vi "WM NH Extreme.vi"(0 "Significant Wave Height":dbl=6.58 min=0.0 step=0.01 format="%.2f", 1 "Sigma A":dbl=0.45 format="%.2f", 3 "Start Freq (Model Scale)":dbl min=0.0 format="%.2f", 4 "Sigma B":dbl=0.15 format="%.2f", 5 "Peak Wave Period":dbl=10.5 min=0.0 step=0.01 format="%.2f", 7 "Number of Frequencies":i32=100 min=2, 9 "Scale Ratio":dbl=15.2 min=0.0 step=0.01 format="%.2f", 11 "P":dbl=4.85 min=-1.0 max=9.0 format="%.2f", 12 "Gamma":dbl=3.95 min=-1.0 max=9.0 format="%.2f", 14 "End Freq (Model Scale)":dbl=100.0 min=0.0 format="%.2f") -> (6 "NH Extreme parameters":T1 {"P" format="%.2f"; "Scale Ratio" format="%.2f"; "Sigma B" format="%.2f"; "Sigma A" format="%.2f"; "Gamma" format="%.2f"; "Sig Wave Period" format="%.2f"; "Sig Wave Height" format="%.2f"}, 10 "Spectral Energy":dbl[](array[numeric]) format="%.2f", 15 "Frequency":dbl[](array[numeric]) caption="Hz" format="%.2f")   [LabVIEW 2012]
panel:
  in  "Boolean":bool
  # "NH Extreme Wave Spectra"
  # "m  (Full Scale)"
  # "s  (Full Scale)"
  # ":1"
  # "Full Scale : Model Scale"
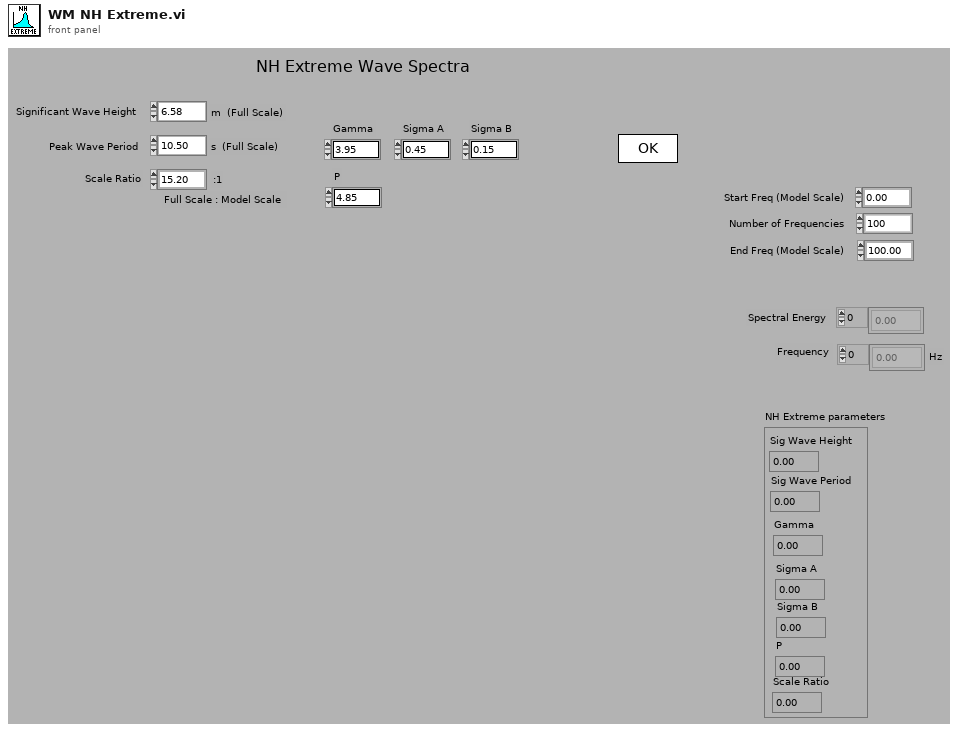
[diagram p1: front panel]
types:
  T1 = cluster{"Sig Wave Height":dbl, "Sig Wave Period":dbl, "Gamma":dbl, "Sigma A":dbl, "Sigma B":dbl, "P":dbl, "Scale Ratio":dbl}
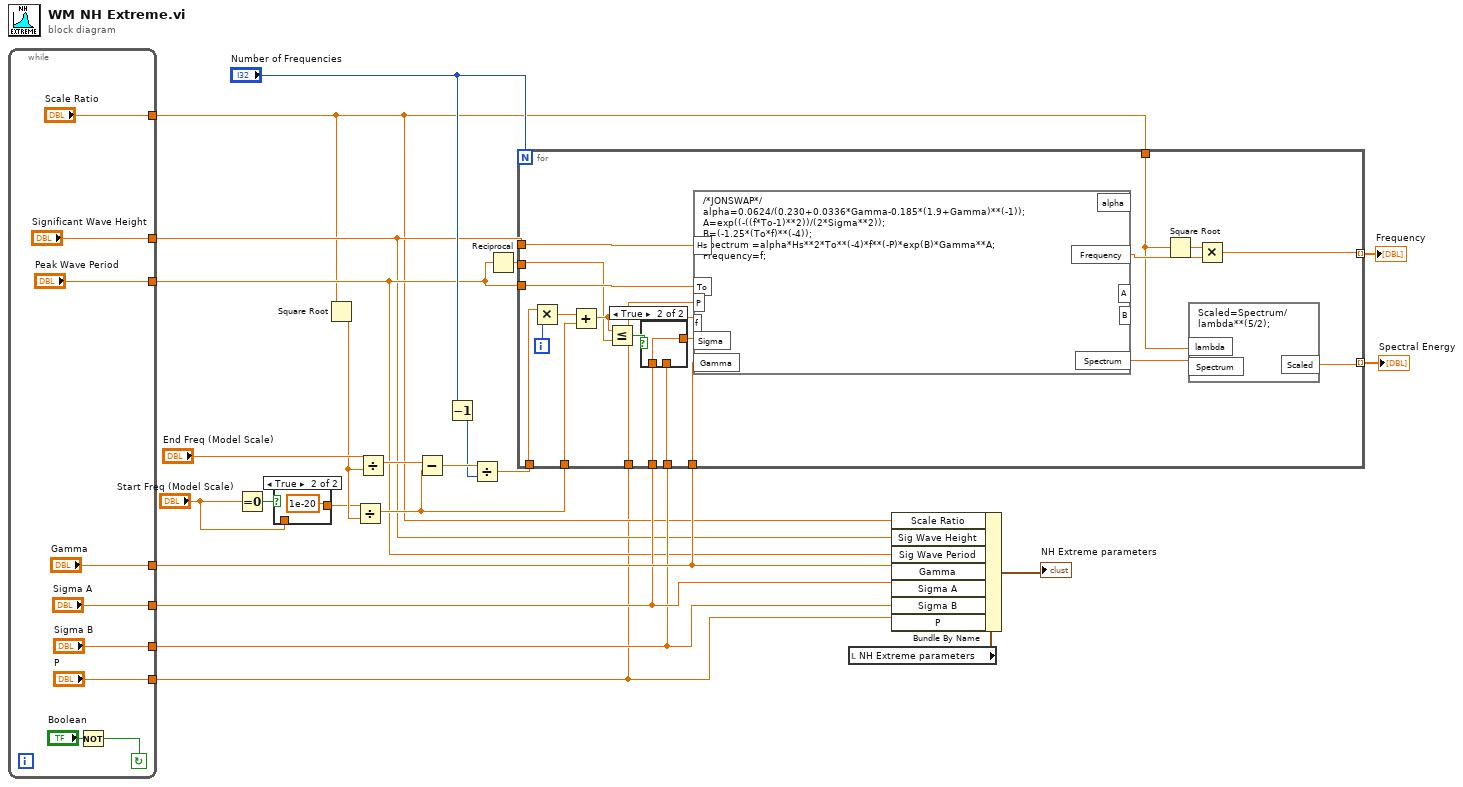
[diagram p0: block diagram]
diagram:
  n1 = while {
    tunnel: ["P"] -> w2
    tunnel: ["Scale Ratio"] -> w3
    tunnel: ["Significant Wave Height"] -> w4
    tunnel: ["Peak Wave Period"] -> w5
    tunnel: ["Sigma B"] -> w6
    tunnel: ["Sigma A"] -> w7
    tunnel: ["Gamma"] -> w8
    stop <- w24 continue-if-true
    n2 = Not(x="Boolean") -> (.not. x?=w24:bool)
  }
  n3 = Equal To 0?(x="Start Freq (Model Scale)") -> (x = 0?=w13:bool)
  n4 = case shown="True" w13 {
    tunnel: [w33 1e-20] -> w11
    tunnel: "Start Freq (Model Scale)" -> [w33 _]
    frame False {
    }
    frame True {
    }
  }
  n5 = Square Root(x=w3) -> (sqrt(x)=w16:dbl)
  n6 = Divide(x=w11, y=w16) -> (x/y=w15:dbl)
  n7 = Divide(x="End Freq (Model Scale)", y=w16) -> (x/y=w14:dbl)
  n8 = Subtract(x=w14, y=w15) -> (x-y=w21:dbl)
  n9 = Decrement(x="Number of Frequencies") -> (x-1=w18:i32)
  n10 = Divide(x=w21, y=w18) -> (x/y=w20:dbl)
  n11 = Reciprocal(x=w5) -> (1/x=w19:dbl)
  n12 = for {
    N: "Number of Frequencies" -> [_]
    tunnel: w4 -> [w43]
    tunnel: w5 -> [w45]
    tunnel: [w38] -> w23 mode=indexing
    tunnel: [w39] -> w1 mode=indexing
    tunnel: w15 -> [w41]
    tunnel: w20 -> [w52]
    tunnel: w19 -> [w44]
    tunnel: w7 -> [w50]
    tunnel: w6 -> [w49]
    tunnel: w8 -> [w48]
    tunnel: w3 -> [w37]
    tunnel: w2 -> [w35]
    i -> [w54]
    n13 = Multiply(x=w52, y=w54) -> (x*y=w42:dbl)
    n14 = Add(x=w42, y=w41) -> (x+y=w46:dbl)
    n15 = Less Or Equal?(x=w46, y=w44) -> (x <= y?=w51:bool)
    n16 = case shown="True" w51 {
      tunnel: w50 -> [_ w56]
      tunnel: w49 -> [w55 _]
      tunnel: [w55 w56] -> w47
      frame False {
      }
      frame True {
      }
    }
    n17 = formula code="/*JONSWAP*/\nalpha=0.0624/(0.230+0.0336*Gamma-0.185*(1.9+Gamma)**(-1));\nA=exp((-((f*To-1)**2))/(2*Sigma**2));\nB=(-1.25*(To*f)**(-4));\nSpectrum =alpha*Hs**2*To**(-4)*f**(-P)*exp(B)*Gamma**A;\nFrequency=f;"("Hs"=w43, "To"=w45, "f"=w46, "Sigma"=w47, "Gamma"=w48, "P"=w35) -> ("Spectrum"=w40:dbl, "Frequency"=w53:dbl)  [unwired: 3 out]
    n18 = Square Root(x=w37) -> (sqrt(x)=w36:dbl)
    n19 = formula code="Scaled=Spectrum/lambda**(5/2);"("lambda"=w37, "Spectrum"=w40) -> ("Scaled"=w39:dbl)
    n20 = Multiply(x=w36, y=w53) -> (x*y=w38:dbl)
  }
  "Spectral Energy" <- w1
  "Frequency" <- w23
  n21 = local read "NH Extreme parameters"() -> (w10:T1)
  n22 = Bundle By Name(cluster=w10, "Scale Ratio"=w3, "Sig Wave Height"=w4, "Sig Wave Period"=w5, "Gamma"=w8, "Sigma A"=w7, "Sigma B"=w6, "P"=w2) -> (→"NH Extreme parameters":T1)
